vi "Intake And Elevator Teleop Control.vi"(8 "D-Pad":T3, 9 "Axes":T1, 10 "Button Cluster":T2) -> ()   [LabVIEW 2017]
uses:
  Common Code/Gamepads/D-Pad.ctl
  Common Code/Gamepads/Button Cluster.ctl
  Common Code/Gamepads/Axes Cluster.ctl
  Common Code/Intake And Elevator States.ctl
  Robot Global Data.vi
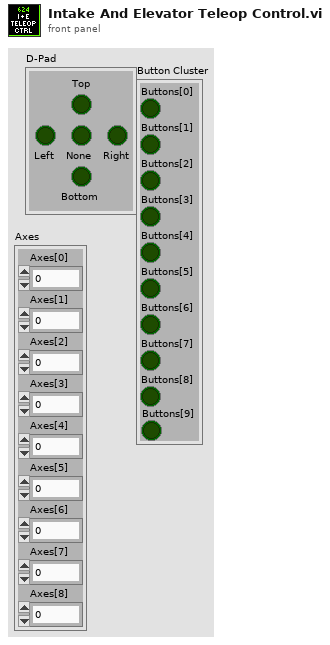
[diagram p1: front panel]
types:
  T1 = typedef "Axes Cluster.ctl" = cluster{"Axes[0]":dbl, "Axes[1]":dbl, "Axes[2]":dbl, "Axes[3]":dbl, "Axes[4]":dbl, "Axes[5]":dbl, "Axes[6]":dbl, "Axes[7]":dbl, "Axes[8]":dbl}
  T2 = typedef "Button Cluster.ctl" = cluster{"Buttons[0]":bool, "Buttons[1]":bool, "Buttons[2]":bool, "Buttons[3]":bool, "Buttons[4]":bool, "Buttons[5]":bool, "Buttons[6]":bool, "Buttons[7]":bool, "Buttons[8]":bool, "Buttons[9]":bool}
  T3 = typedef "D-Pad.ctl" = cluster{"Top":bool, "Bottom":bool, "None":bool, "Right":bool, "Left":bool}
  T4 = typedef "Intake And Elevator States.ctl" = enum16{"Idle", "Pick Up Cube", "Switch", "Scale ", "Endgame"}
  T5 = typedef "Intake And Elevator Command Cluster.ctl" = cluster{"States ":T4, "Grab?":bool, "Drop?":bool, "Mode":T6, "Override Lift":bool, "Override Lift":dbl, "High?":bool}
  T6 = typedef "Intake and Elevator Mode.ctl" = enum16{"Auto", "Not Auto"}
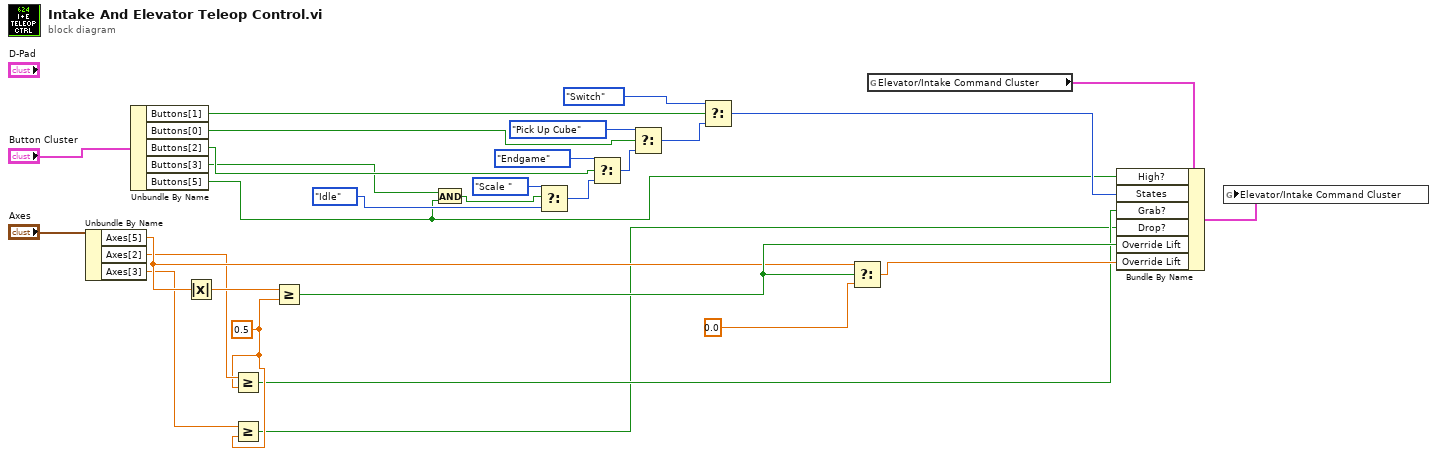
[diagram p0: block diagram]
diagram:
  w6 = 0.5
  n1 = Unbundle By Name("Axes") -> ("Axes[5]"=w14:dbl, "Axes[2]"=w8:dbl, "Axes[3]"=w7:dbl)
  n2 = Unbundle By Name("Button Cluster") -> ("Buttons[1]"=w11:bool, "Buttons[0]"=w24:bool, "Buttons[2]"=w20:bool, "Buttons[3]"=w2:bool, "Buttons[5]"=w1:bool)
  n3 = Absolute Value(x=w14) -> (abs(x)=w16:dbl)
  n4 = Greater Or Equal?(x=w8, y=w6) -> (x >= y?=w5:bool)
  n5 = Greater Or Equal?(x=w7, y=w6) -> (x >= y?=w4:bool)
  n6 = Greater Or Equal?(x=w16, y=w6) -> (x >= y?=w15:bool)
  n7 = And(x=w2, y=w1) -> (x .and. y?=w3:bool)
  n8 = Select(t=Intake_And_Elevator_States."Scale " ("States"), s=w3, f=Intake_And_Elevator_States."Idle" ("States")) -> (s? t:f=w18:T4)
  n9 = Select(t=Intake_And_Elevator_States."Endgame" ("States"), s=w20, f=w18) -> (s? t:f=w23:T4)
  n10 = Select(t=Intake_And_Elevator_States."Pick Up Cube" ("States"), s=w24, f=w23) -> (s? t:f=w22:T4)
  n11 = Select(t=Intake_And_Elevator_States."Switch" ("States"), s=w11, f=w22) -> (s? t:f=w10:T4)
  n12 = Select(t=w14, s=w15, f=0.0) -> (s? t:f=w12:dbl)
  n13 = global read "Robot Global Data.vi" "Elevator/Intake Command Cluster"() -> (w28:T5)
  n14 = Bundle By Name(cluster=w28, "High?"=w1, "States"=w10, "Grab?"=w5, "Drop?"=w4, "Override Lift"=w15, "Override Lift"=w12) -> (w27:T5)
  n15 = global write "Robot Global Data.vi" "Elevator/Intake Command Cluster"(w27) -> ()
